vi "PhotonPNPResult_IsPresent.vi"(11 "PhotonPNPResult":T1={"IsPresent"=FALSE, "bestReprojErr"=0.0, "altReprojErr"=0.0, "ambiguity"=0.0, "Best"={"TRANSLATION3D"={"X"=0.0, "Y"=0.0, "Z"=0.0}, "ROTATION3D"={"Q_quaternion"={"R"=1.0, "V"=[0.0, 0.0, 0.0]}}, "XF"=FALSE}, "Alt"={"TRANSLATION3D"={"X"=0.0, "Y"=0.0, "Z"=0.0}, "ROTATION3D"={"Q_quaternion"={"R"=1.0, "V"=[0.0, 0.0, 0.0]}}, "XF"=FALSE}} {"Alt"."TRANSLATION3D"."Z" format="%14.3f"; "Alt"."TRANSLATION3D"."Y" format="%14.3f"; "Alt"."TRANSLATION3D"."X" format="%14.3f"; "Best"."TRANSLATION3D"."Z" format="%14.3f"; "Best"."TRANSLATION3D"."Y" format="%14.3f"; "Best"."TRANSLATION3D"."X" format="%14.3f"}) -> (3 "IsPresent":bool)   [LabVIEW 2019, in "PhotonVisionLib.lvlib"]
doc: "Determines if PNP Result is present.\n\nInputs:\n - PhotonPNPResult -- PhotonPNPResult cluster.\n\nOutputs:\n - IsPresent -- Returns TRUE, if a PNP Result is present."
uses:
  TypeDef/PhotonPNPResultType.ctl
  <vilib>/Rock Robotics/WPI/ThirdParty/JAS_Junk/TrajLib/TypeDef/TRANSFORM3D.ctl
  <vilib>/Rock Robotics/WPI/ThirdParty/JAS_Junk/TrajLib/TypeDef/TRANSLATION3D.ctl
  <vilib>/Rock Robotics/WPI/ThirdParty/JAS_Junk/TrajLib/TypeDef/ROTATION3D.ctl
  <vilib>/Rock Robotics/WPI/ThirdParty/JAS_Junk/TrajLib/TypeDef/QUATERNION.ctl
  <vilib>/Rock Robotics/WPI/ThirdParty/JAS_Junk/TrajLib/VI/Transform3d_GetTranslation3d.vi
  <vilib>/Rock Robotics/WPI/ThirdParty/JAS_Junk/TrajLib/VI/Transform3d_GetRotation3d.vi
  <vilib>/Rock Robotics/WPI/ThirdParty/JAS_Junk/TrajLib/VI/Rotation3d_Equals.vi
  <vilib>/Rock Robotics/WPI/ThirdParty/JAS_Junk/TrajLib/VI/Translation3d_Equals.vi
  <vilib>/Rock Robotics/WPI/ThirdParty/JAS_Junk/TrajLib/VI/Rotation3d_GetQuaterion.vi
  <vilib>/Rock Robotics/WPI/ThirdParty/JAS_Junk/TrajLib/VI/Quaternion_Equals.vi
  <vilib>/Rock Robotics/WPI/ThirdParty/JAS_Junk/TrajLib/VI/Quaternion_Get_Vect.vi
  <vilib>/Rock Robotics/WPI/ThirdParty/JAS_Junk/TrajLib/VI/Quaternion_Get_W.vi
  PhotonVisionLib.lvlib
  <vilib>/Rock Robotics/WPI/ThirdParty/JAS_Junk/TrajLib/Trajectory_Library.lvlib
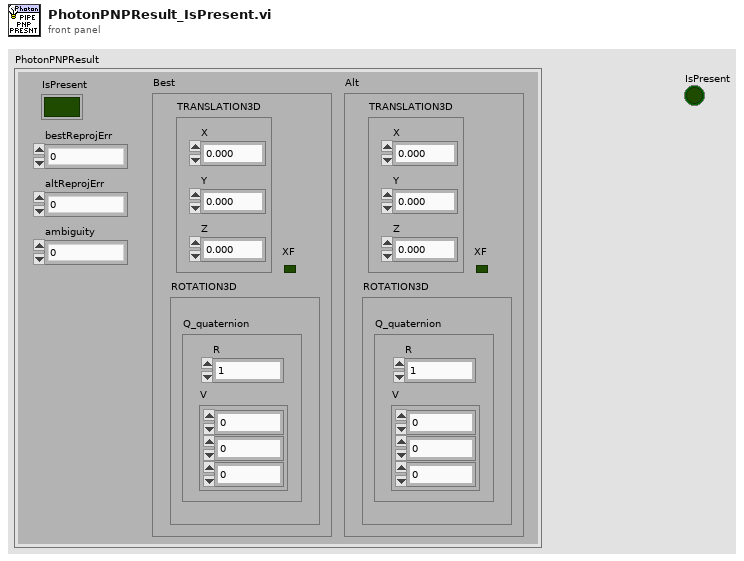
[diagram p1: front panel]
types:
  T1 = typedef "PhotonVisionLib.lvlib/PhotonPNPResultType.ctl" = cluster{"IsPresent":bool, "bestReprojErr":dbl, "altReprojErr":dbl, "ambiguity":dbl, "Best":T2, "Alt":T2}
  T2 = typedef "Trajectory_Library.lvlib/TRANSFORM3D.ctl" = cluster{"TRANSLATION3D":T3, "ROTATION3D":T4, "XF":bool}
  T3 = typedef "Trajectory_Library.lvlib/TRANSLATION3D.ctl" = cluster{"X":dbl, "Y":dbl, "Z":dbl}
  T4 = typedef "Trajectory_Library.lvlib/ROTATION3D.ctl" = cluster{"Q_quaternion":T5}
  T5 = typedef "Trajectory_Library.lvlib/QUATERNION.ctl" = cluster{"R":dbl, "V":dbl[]}
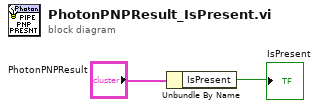
[diagram p0: block diagram]
diagram:
  n1 = Unbundle By Name("PhotonPNPResult") -> ("IsPresent"=→"IsPresent":bool)
